vi "Get Result.vi"(8 "error in (no error)":errorcluster, 11 "Instrument Recorder in":refnum<class "Instrument Recorder.lvclass">) -> (0 "error out":errorcluster, 2 "Result":refnum<class "Acquired Result.lvclass">, 3 "Instrument Recorder out":refnum<class "Instrument Recorder.lvclass">)   [LabVIEW 2015, in "Instrument Recorder.lvclass"]
uses:
  Instrument Recorder.lvclass
  Results/Acquired Result/Acquired Result.lvclass
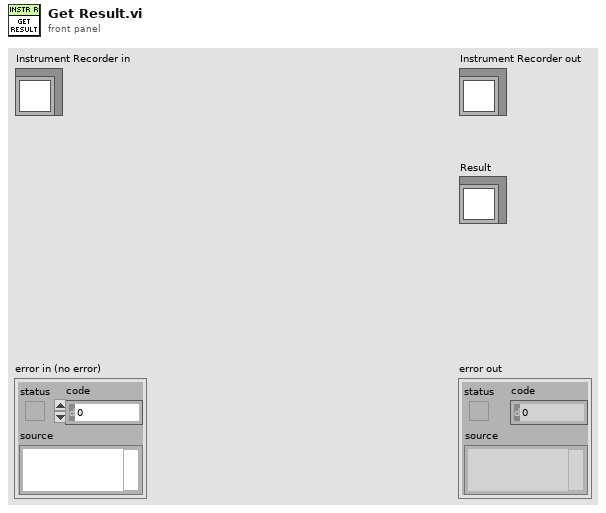
[diagram p1: front panel]
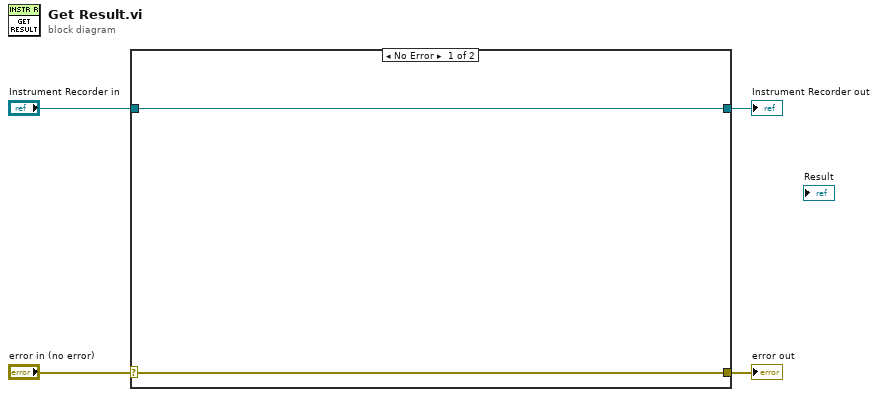
[diagram p0: block diagram]
diagram:
  n1 = case shown="No Error" "error in (no error)" {
    selector: "error in (no error)" -> [w5 w8]
    tunnel: [w5 w8] -> w3
    tunnel: [w6 w7] -> w1
    tunnel: "Instrument Recorder in" -> [w6 w7]
    frame No Error {
    }
    frame Error {
    }
  }
  "error out" <- w3
  "Instrument Recorder out" <- w1
